vi "Set QWTB Path.vi"(6 "Backend engine":T1, 8 "error in":errorcluster, 11 "QWTB Folder Path":path=path "") -> (0 "error out":errorcluster)   [LabVIEW 2013]
doc: "Set matlab working path to qwtb directory."
uses:
  TD Backend Engine.ctl
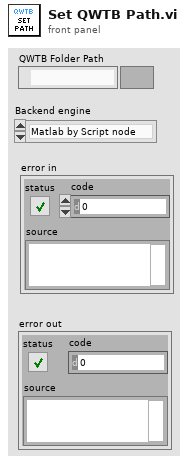
[diagram p1: front panel]
types:
  T1 = typedef "TD Backend Engine.ctl" = enum16{"Matlab by Script node", "GNU Octave by GOLPI"}
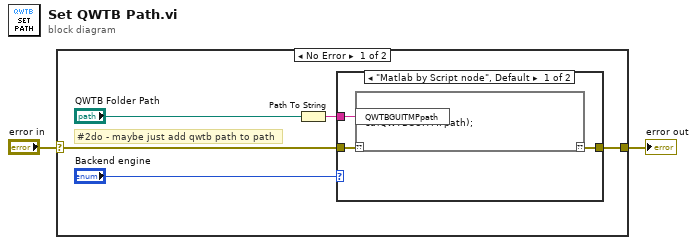
[diagram p0: block diagram]
diagram:
  n1 = case shown="No Error" "error in" {
    selector: "error in" -> [w6 w12]
    tunnel: [w7 w12] -> w2
    frame No Error {
      # "#2do - maybe just add qwtb path to path"
      n2 = Path To String(path="QWTB Folder Path") -> (string=w5:string)
      n3 = case shown="\"Matlab by Script node\", Default" "Backend engine" {
        tunnel: [w10 w11] -> w7
        tunnel: w6 -> [w9 w11]
        tunnel: w5 -> [w8 _]
        frame "Matlab by Script node", Default {
          n4 = script code="cd(QWTBGUITMPpath);"("??"=w9, "QWTBGUITMPpath"=w8) -> ("??"=w10:errorcluster)
        }
        frame "GNU Octave by GOLPI" {
          # "#2do"
        }
      }
    }
    frame Error {
    }
  }
  "error out" <- w2
